vi "NewTestSkill.vi"(9 "NewTestSkill.lvclass":refnum<class "NewTestSkill.lvclass">, 10 "Robot":refnum<class "Robot.lvclass">) -> (1 "NewTestSkill.lvclass 2":refnum<class "NewTestSkill.lvclass">, 2 "Robot out":refnum<class "Robot.lvclass">)   [LabVIEW 2022 SP3, in "NewTestSkill.lvclass"]
uses:
  NewTestSkill.lvclass
  Robot_class/Robot.lvclass
  Robot_class/Robot.lvclass/Robot.ctl
  Robot_class/Write dest_x.vi
  Robot_class/Write dest_y.vi
  Robot_class/Write dest_orientation.vi
panel:
  out "error out":errorcluster
  in  "error in (no error)":errorcluster
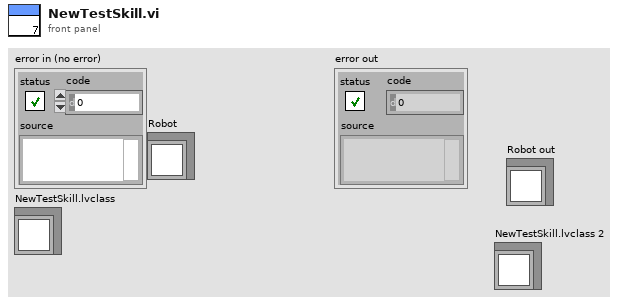
[diagram p1: front panel]
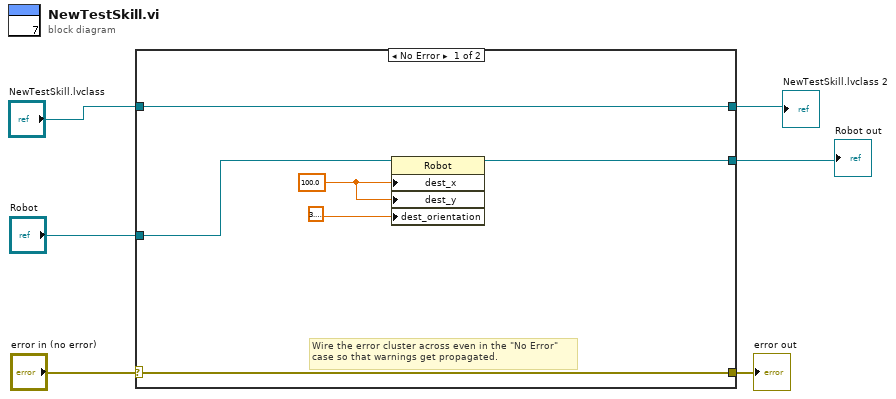
[diagram p0: block diagram]
diagram:
  n1 = case shown="No Error" "error in (no error)" {
    selector: "error in (no error)" -> [w12 w15]
    tunnel: [w12 w15] -> w5
    tunnel: "Robot" -> [w11 w14]
    tunnel: [w10 w14] -> w3
    tunnel: "NewTestSkill.lvclass" -> [w7 w13]
    tunnel: [w7 w13] -> w1
    frame No Error {
      w9 = 100.0 ("dest_x")
      # "Wire the error cluster across even in the \"No Error\"\ncase so that warnings get propagated."
      n2 = property class="Robot"(reference=w11, "dest_x"=w9, "dest_y"=w9, "dest_orientation"=3.141592653589793) -> (reference out=w10:refnum<class "Robot.lvclass">)  [unwired: 1 in, 1 out]
    }
    frame Error {
    }
  }
  "error out" <- w5
  "Robot out" <- w3
  "NewTestSkill.lvclass 2" <- w1
